vi "SetAmPhase.vi"(8 "error in (no error)":errorcluster, 9 "fclk (MHz)":dbl=10.0 format="%#_13g", 10 "Am freq [kHz]":dbl=10.0, 11 "FpgaRef5782 in":refnum<class "FpgaRef5782.lvclass">) -> (0 "error out":errorcluster, 3 "FpgaRef5782 out":refnum<class "FpgaRef5782.lvclass">)   [LabVIEW 2018, in "FpgaRef5782.lvclass"]
uses:
  FpgaRef5782.lvclass
  FpgaRef5782.lvclass/FpgaRef5782.ctl
  <vilib>/Utility/error.llb/Error Cluster From Error Code.vi
  <vilib>/rvi/errors/niLvFpgaAdjustHostInterfaceError.vi
  <vilib>/rvi/interface/nirviReadWriteControl/nirviReadWriteControl.xnode
  5782 FPGA ref.ctl
  NiFpgaLv.dll
  <vilib>/rvi/interface/Simulation/niFpgaSimulationCallBeginRW.vi
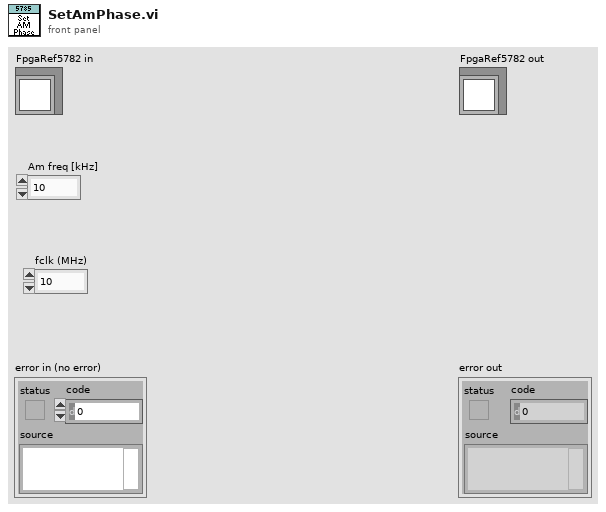
[diagram p1: front panel]
types:
  T1 = typedef "5782 FPGA ref.ctl" = refnum<k20>
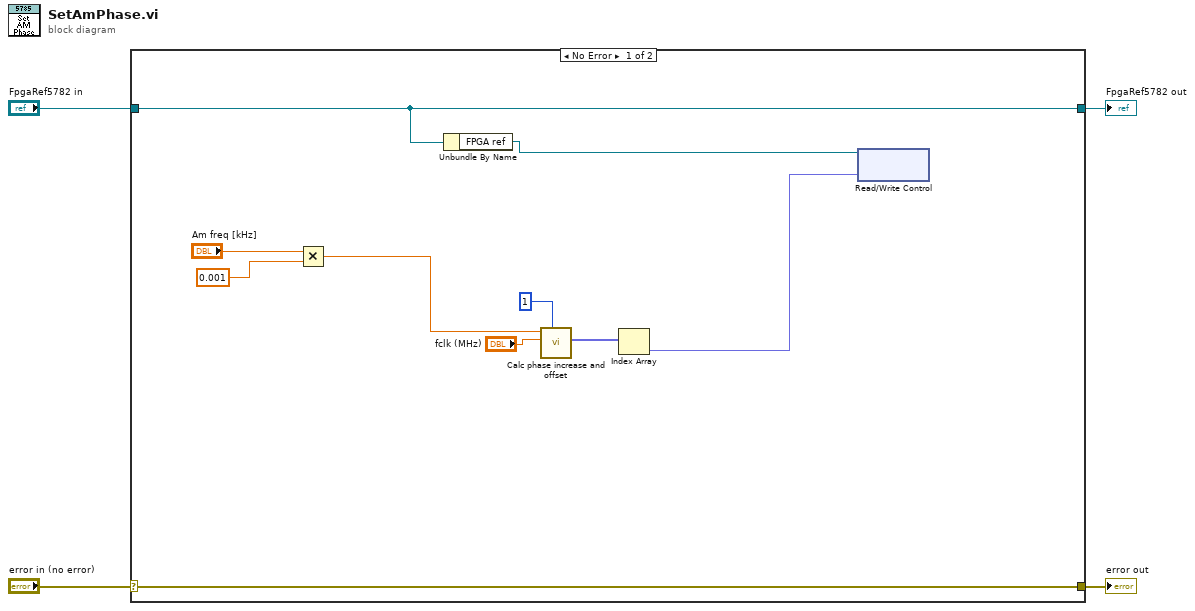
[diagram p0: block diagram]
diagram:
  n1 = case shown="No Error" "error in (no error)" {
    selector: "error in (no error)" -> [w14 w16]
    tunnel: [w14 w16] -> w3
    tunnel: [w13 w15] -> w1
    tunnel: "FpgaRef5782 in" -> [w13 w15]
    frame No Error {
      n2 = Multiply(x="Am freq [kHz]", y=0.001) -> (x*y=w6:dbl)
      n3 = Unbundle By Name(w13) -> ("FPGA ref"=w12:T1)
      n4 = call "Calc phase increase and offset.vi"("# of DDS"=1, "fclk (MHz)"="fclk (MHz)", "f_generated (MHz)"=w6) -> ("Phase out"=w7:fxp<+,64,64>[])  [unwired: 6 in, 2 out]
      n5 = Index Array(array=w7) -> (element=w5:fxp<+,64,64>)  [unwired: 1 in]
      n6 = xnode "Read/Write Control"("FPGA VI Reference In"=w12, "AM phase"=w5) -> ()  [unwired: 1 in, 2 out]
    }
    frame Error {
    }
  }
  "error out" <- w3
  "FpgaRef5782 out" <- w1
